vi "Register gRPC Methods.vi"(8 "error in (no error)":errorcluster, 11 "gRPC service in":refnum<class "ExamplePluginOOBService.lvclass">) -> (0 "error out":errorcluster, 3 "gRPC service out":refnum<class "ExamplePluginOOBService.lvclass">)   [LabVIEW 2025, in "ExamplePluginOOBService_server.lvlib" / "ExamplePluginOOBService.lvclass"]
uses:
  ExamplePluginOOBService.lvclass
  typeDefs/Server Internal UEs.ctl
  typeDefs/Server Internal Message.ctl
  typeDefs/Server gRPC UEs.ctl
  <vilib>/gRPC/LabVIEW gRPC Library/Server API/typeDefs/gRPCId Cluster.ctl
  <vilib>/gRPC/LabVIEW gRPC Library/Shared/grpcId.ctl
  ExamplePluginOOBService.lvclass/ExamplePluginOOBService.ctl
  <vilib>/gRPC/LabVIEW gRPC Library/grpc-lvsupport-release.lvlib
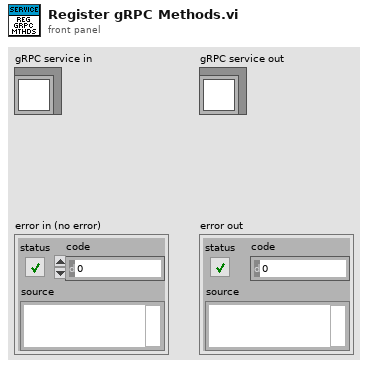
[diagram p1: front panel]
types:
  T1 = typedef "ExamplePluginOOBService_server.lvlib/ExamplePluginOOBService.lvclass/Server gRPC UEs.ctl" = cluster{"ExamplePluginOOBService Execute gRPC UE":refnum<user-event>, "ExamplePluginOOBService Pause gRPC UE":refnum<user-event>, "ExamplePluginOOBService Resume gRPC UE":refnum<user-event>, "ExamplePluginOOBService Export gRPC UE":refnum<user-event>}
  T2 = typedef "ExamplePluginOOBService_server.lvlib/ExamplePluginOOBService.lvclass/Server Internal UEs.ctl" = cluster{"ExamplePluginOOBService Execute Internal UE":refnum<user-event>, "ExamplePluginOOBService Pause Internal UE":refnum<user-event>, "ExamplePluginOOBService Resume Internal UE":refnum<user-event>, "ExamplePluginOOBService Export Internal UE":refnum<user-event>}
  T3 = typedef "grpc-lvsupport-release.lvlib/grpcId.ctl" = u64
  T4 = typedef "ExamplePluginOOBService_server.lvlib/ExamplePluginOOBService.lvclass/Server Internal Message UE.ctl" = refnum<user-event>
  T5 = typedef "grpc-lvsupport-release.lvlib/gRPCId Cluster UE.ctl" = refnum<user-event>
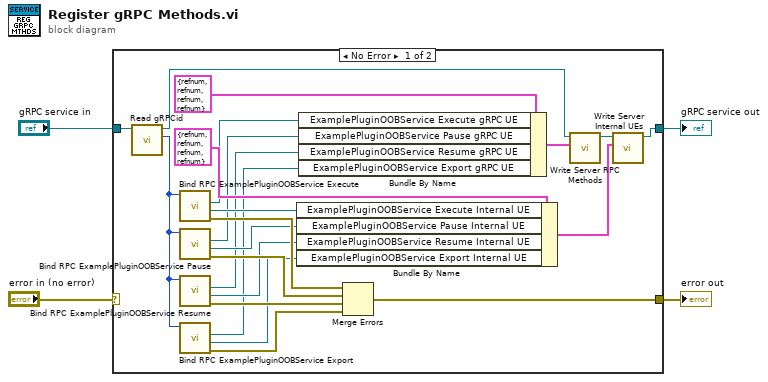
[diagram p0: block diagram]
diagram:
  n1 = case shown="No Error" "error in (no error)" {
    selector: "error in (no error)" -> [_ w27]
    tunnel: "gRPC service in" -> [w18 w28]
    tunnel: [w26 w27] -> w3
    tunnel: [w25 w28] -> w2
    frame No Error {
      n2 = call-dynamic "Read gRPCid.vi"("gRPC service in"=w18) -> ("gRPCid"=w17:T3, "gRPC service out"=w19:refnum<class "ExamplePluginOOBService.lvclass">)  [unwired: 8 in, 1 out]
      n3 = call "Bind RPC ExamplePluginOOBService Execute.vi"("gRPCid server in"=w17) -> ("error out"=w16:errorcluster, "ExamplePluginOOBService Execute Internal UE"=w14:T4, "ExamplePluginOOBService Execute gRPC UE"=w15:T5)  [unwired: 7 in, 1 out]
      n4 = call "Bind RPC ExamplePluginOOBService Pause.vi"("gRPCid server in"=w17) -> ("error out"=w13:errorcluster, "ExamplePluginOOBService Pause Internal UE"=w11:T4, "ExamplePluginOOBService Pause gRPC UE"=w12:T5)  [unwired: 7 in, 1 out]
      n5 = call "Bind RPC ExamplePluginOOBService Resume.vi"("gRPCid server in"=w17) -> ("error out"=w10:errorcluster, "ExamplePluginOOBService Resume Internal UE"=w8:T4, "ExamplePluginOOBService Resume gRPC UE"=w9:T5)  [unwired: 7 in, 1 out]
      n6 = call "Bind RPC ExamplePluginOOBService Export.vi"("gRPCid server in"=w17) -> ("error out"=w7:errorcluster, "ExamplePluginOOBService Export Internal UE"=w5:T4, "ExamplePluginOOBService Export gRPC UE"=w6:T5)  [unwired: 7 in, 1 out]
      n7 = Bundle By Name ("Bundle Internal UEs")(cluster=T2 {"ExamplePluginOOBService Execute Internal UE"=refnum, "ExamplePluginOOBService Pause Internal UE"=refnum, "ExamplePluginOOBService Resume Internal UE"=refnum, "ExamplePluginOOBService Export Internal UE"=refnum} ("Server Internal UEs"), "ExamplePluginOOBService Execute Internal UE"=w14, "ExamplePluginOOBService Pause Internal UE"=w11, "ExamplePluginOOBService Resume Internal UE"=w8, "ExamplePluginOOBService Export Internal UE"=w5) -> (w24:T2)
      n8 = Bundle By Name ("Bundle gRPC UEs")(cluster=T1 {"ExamplePluginOOBService Execute gRPC UE"=refnum, "ExamplePluginOOBService Pause gRPC UE"=refnum, "ExamplePluginOOBService Resume gRPC UE"=refnum, "ExamplePluginOOBService Export gRPC UE"=refnum} ("gRPC Server Method Events"), "ExamplePluginOOBService Execute gRPC UE"=w15, "ExamplePluginOOBService Pause gRPC UE"=w12, "ExamplePluginOOBService Resume gRPC UE"=w9, "ExamplePluginOOBService Export gRPC UE"=w6) -> (w21:T1)
      n9 = Merge Errors(w16, w13, w10, w7) -> (w26:errorcluster)
      n10 = call "Write Server RPC Methods.vi"("Server RPC Methods"=w21, "gRPC service in"=w19) -> ("gRPC service out"=w22:refnum<class "ExamplePluginOOBService.lvclass">)  [unwired: 8 in, 1 out]
      n11 = call "Write Server Internal UEs.vi"("Server Internal UEs"=w24, "gRPC service in"=w22) -> ("gRPC service out"=w25:refnum<class "ExamplePluginOOBService.lvclass">)  [unwired: 8 in, 1 out]
    }
    frame Error {
    }
  }
  "error out" <- w3
  "gRPC service out" <- w2
